vi "Deploy to Last Target.vi"(8 "error in (no error)":errorcluster, 10 "Source Via":path, 11 "GVIWebProcessorApp in":refnum<class "GVIWebProcessorApp.lvclass">) -> (0 "error out":errorcluster, 3 "GVIWebProcessorApp out":refnum<class "GVIWebProcessorApp.lvclass">)   [LabVIEW 2020, in "PicoG-Processor.lvlib" / "GVIWebProcessorApp.lvclass"]
uses:
  GVIWebProcessorApp.lvclass
  Builds/picoG/ppl/PicoG-Core.lvlibp/PicoG-Processor/PicoG-Core/PlatformPluginManager/PlatformPluginManager.lvclass
  Builds/picoG/ppl/PicoG-Core.lvlibp/PicoG-Processor/PicoG-Core/DeployPlatform/DeployPlatform.lvclass
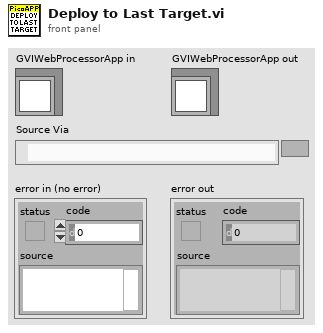
[diagram p1: front panel]
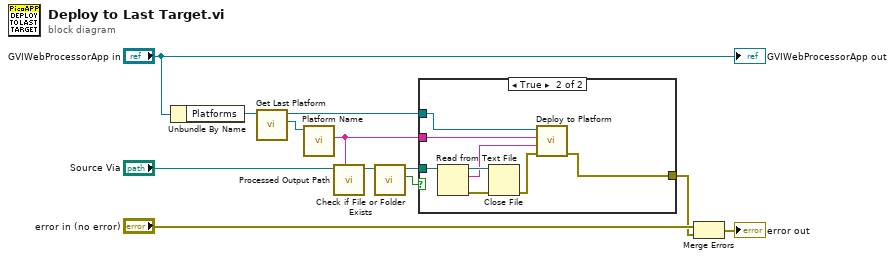
[diagram p0: block diagram]
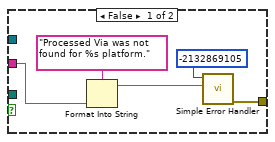
[diagram p2: hidden frame]
diagram:
  n1 = Unbundle By Name("GVIWebProcessorApp in") -> ("Platforms"=w11:refnum<class "PlatformPluginManager.lvclass">)
  n2 = call "Get Last Platform.vi"("TargetPluginManager in"=w11) -> ("Last Platform"=w10:refnum<class "DeployPlatform.lvclass">, "TargetPluginManager out"=w1:refnum<class "PlatformPluginManager.lvclass">)  [unwired: 8 in, 1 out]
  n3 = call-dynamic "Platform Name.vi"("DeployTarget in"=w10) -> ("Platform Name"=w2:string)  [unwired: 8 in, 2 out]
  n4 = call "Processed Output Path.vi"("Platform"=w2, "Source Via Path"="Source Via") -> ("Processed Output Path"=w7:path)  [unwired: 8 in, 1 out]
  n5 = call <vilib>:"Check if File or Folder Exists.vi"("path"=w7) -> ("file or folder exists?"=w6:bool, "dup path"=w5:path)  [unwired: 8 in, 1 out]
  n6 = case shown="True" w6 {
    tunnel: w5 -> [_ w25]
    tunnel: [w16 w18] -> w3
    tunnel: w2 -> [w14 w21]
    tunnel: w1 -> [_ w20]
    frame False {
      n7 = Format Into String(format string="Processed Via was not found for %s platform.", w14) -> (resulting string=w13:string)  [unwired: 2 in, 1 out]
      n8 = call <vilib>:"Simple Error Handler.vi"("error code (no error:0)"=-2132869105, "error source (\" \")"=w13) -> ("error out"=w16:errorcluster)  [unwired: 3 in, 4 out]
    }
    frame True {
      n9 = Read from Text File(file (use dialog)=w25) -> (refnum out=w24:refnum<file>, text=w22:string, error out=w23:errorcluster)  [unwired: 3 in, 1 out]
      n10 = Close File(refnum=w24, error in=w23) -> (error out=w19:errorcluster)  [unwired: 1 out]
      n11 = call "Deploy to Platform.vi"("error in (no error)"=w19, "Processed VIA"=w22, "Platform"=w21, "TargetPluginManager in"=w20) -> ("error out"=w18:errorcluster)  [unwired: 3 in, 4 out]
    }
  }
  n12 = Merge Errors("error in (no error)", w3) -> (→"error out":errorcluster)
  "GVIWebProcessorApp out" <- "GVIWebProcessorApp in"
